vi "_back_view.vi"(8 "error in (no error)":errorcluster, 9 "other":refnum<class "Value.lvclass">, 10 "prev":refnum<class "Value.lvclass">, 11 "IN":refnum<class "Value.lvclass">) -> (0 "error out":errorcluster, 1 "other":refnum<class "Value.lvclass">, 2 "prev":refnum<class "Value.lvclass">, 3 "Value out":refnum<class "Value.lvclass">, 4 "OTHER":T1={"Value"=0.0, "grad"=0.0, "label"="", "operation"=enum."add", "serial"=0}, 5 "IN":T1={"Value"=0.0, "grad"=0.0, "label"="", "operation"=enum."add", "serial"=0}, 6 "PREV":T1={"Value"=0.0, "grad"=0.0, "label"="", "operation"=enum."add", "serial"=0})   [LabVIEW 2023, in "LabGRAD.lvlib" / "Value.lvclass"]
uses:
  Value.lvclass
  Value.lvclass/Value.ctl
  UiObjects/numeric value control.ctl
  UiObjects/UiObjects.lvclass
  UiObjects/string control.ctl
  operation.ctl
  value view.ctl
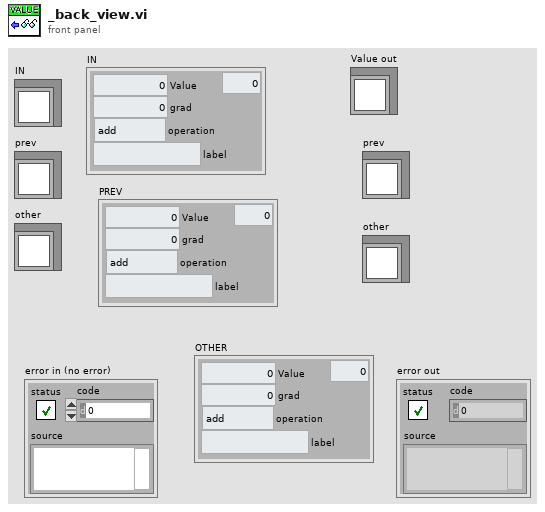
[diagram p1: front panel]
types:
  T1 = typedef "LabGRAD.lvlib/Value.lvclass/value view.ctl" = cluster{"Value":T2, "grad":T2, "label":T3, "operation":T4, "serial":u32}
  T2 = typedef "UiObjects.lvlib/UiObjects.lvclass/numeric value control.ctl" = dbl
  T3 = typedef "UiObjects.lvlib/UiObjects.lvclass/string control.ctl" = string
  T4 = typedef "LabGRAD.lvlib/Value.lvclass/operation.ctl" = enum16{"nop", "add", "subtract", "power", "multiply", "divide", "tanh"}
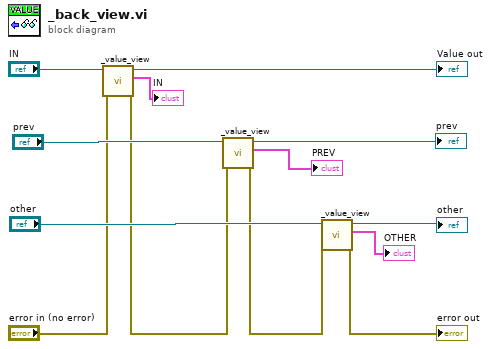
[diagram p0: block diagram]
diagram:
  n1 = call "_value_view.vi"("error in (no error)"="error in (no error)", "Value in"="IN") -> ("error out"=w5:errorcluster, "Val View"=→"IN":T1, "Value out"=→"Value out":refnum<class "Value.lvclass">)  [unwired: 7 in]
  n2 = call "_value_view.vi"("error in (no error)"=w5, "Value in"="prev") -> ("error out"=w4:errorcluster, "Val View"=→"PREV":T1, "Value out"=→"prev":refnum<class "Value.lvclass">)  [unwired: 7 in]
  n3 = call "_value_view.vi"("error in (no error)"=w4, "Value in"="other") -> ("error out"=→"error out":errorcluster, "Val View"=→"OTHER":T1, "Value out"=→"other":refnum<class "Value.lvclass">)  [unwired: 7 in]
